vi "AccumulateHistogram.vi"(8 "Array in":i32[](array[numeric]), 11 "Histogram graph in":T1) -> (0 "Array out":i32[](array[numeric]), 3 "Histogram graph out":T1)   [LabVIEW 2012]
panel:
  out "size(s) 3":i32
  out "size(s) 2":i32
  out "size(s)":i32
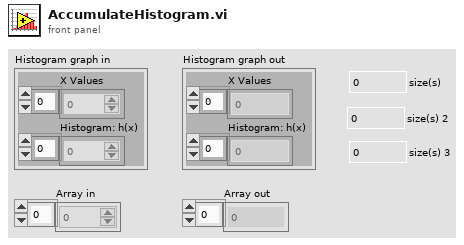
[diagram p1: front panel]
types:
  T1 = cluster{"X Values":dbl[], "Histogram: h(x)":i32[]}
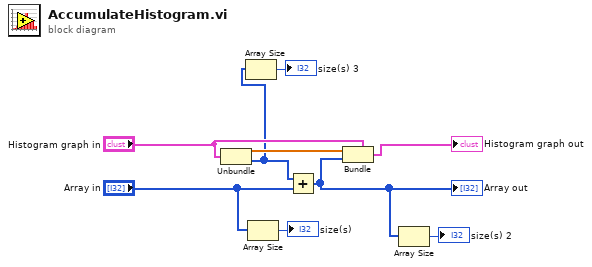
[diagram p0: block diagram]
diagram:
  n1 = Unbundle("Histogram graph in") -> ("X Values"=w8:dbl[], "Histogram: h(x)"=w1:i32[])
  n2 = Array Size(array=w1) -> (size(s)=→"size(s) 3":i32)
  n3 = Array Size(array="Array in") -> (size(s)=→"size(s)":i32)
  n4 = Add(x=w1, y="Array in") -> (x+y=w3:i32[])
  "Array out" <- w3
  n5 = Bundle(cluster="Histogram graph in", "X Values"=w8, "Histogram: h(x)"=w3) -> (→"Histogram graph out":T1)
  n6 = Array Size(array=w3) -> (size(s)=→"size(s) 2":i32)
